vi "Load IV Data.vi"(7 "Other channels":string[](array[string]), 8 "error in":errorcluster, 9 "All scans":refnum<vi>, 10 "Scan numbers":i32[](array[numeric])=[0], 11 "File Path":path=path "U:/My Documents/Projects/Eremets/NV/IV/Data/August_2022/080922/m009_080922.tdms") -> (0 "error out":errorcluster, 1 "dIdV":dbl[](array[numeric]) format="%#_6p", 2 "V":dbl[](array[numeric]), 3 "I":dbl[](array[numeric]), 4 "Other values":string[](array[string]), 5 "Number of scans":i32)   [LabVIEW 2021]
panel:
  out "Numeric 2":i32
  out "Numeric":i32
  out "group names":string[](array[string])
  out "f 2":cluster{dbl[], dbl[]}(graph)
  out "All scans":cluster{dbl[], dbl[]}[](graph)
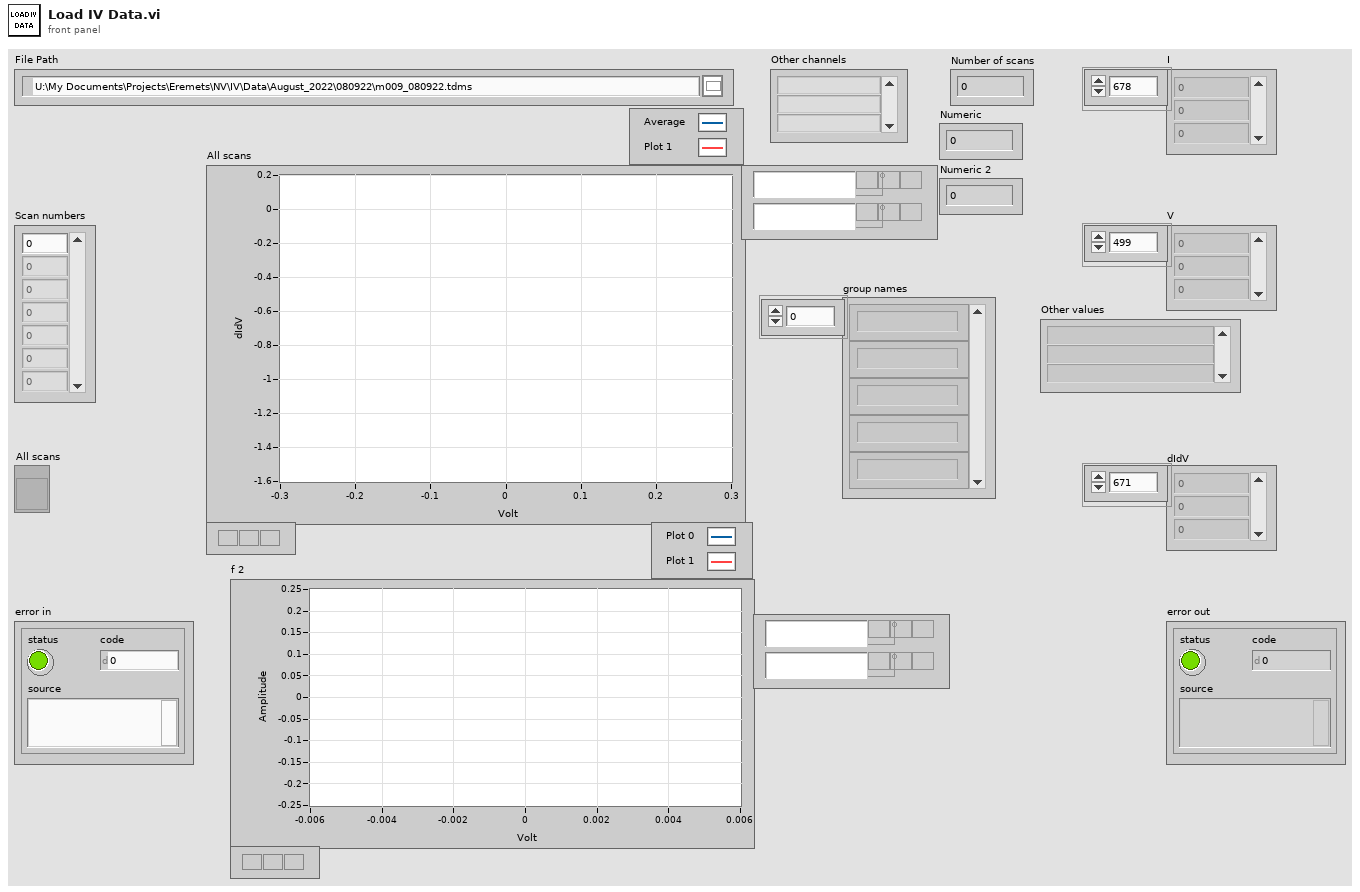
[diagram p1: front panel]
types:
  T1 = enum16{"open", "open or create", "create or replace", "create", "open (read-only)"}
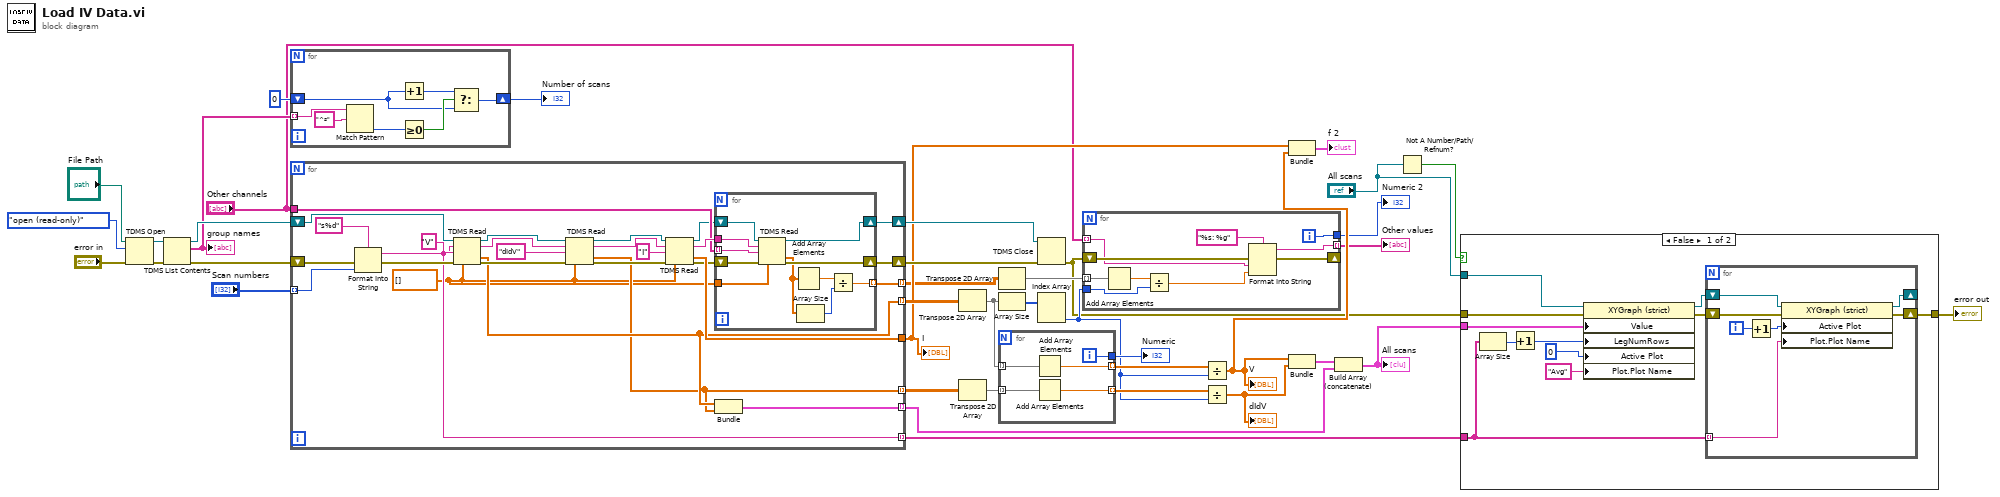
[diagram p0: block diagram]
diagram:
  n1 = TDMS Open(8:"error in", 10:T1."open (read-only)" ("operation (0:open)"), 11:"File Path") -> (0:w18:errorcluster, 3:w20:refnum<k34>)  [unwired: 4 in]
  n2 = TDMS List Contents(4:w18, 7:w20) -> (0:w17:errorcluster, 2:w16:string[], 3:w19:refnum<k34>)  [unwired: 1 in, 1 out]
  "group names" <- w16
  n3 = for {
    tunnel: w16 -> [w46] mode=indexing
    shift-right: [w40] -> w14
    shift-left: 0 -> [w41]
    n4 = Match Pattern(string=w46, regular expression="^s") -> (offset past match=w44:i32)  [unwired: 1 in, 3 out]
    n5 = Increment(x=w41) -> (x+1=w42:i32)
    n6 = Greater Or Equal To 0?(x=w44) -> (x >= 0?=w43:bool)
    n7 = Select(t=w42, s=w43, f=w41) -> (s? t:f=w40:i32)
  }
  "Number of scans" <- w14
  n8 = for {
    shift-right: [w51] -> w35
    shift-left: w17 -> [w64]
    tunnel: [w57] -> w33 mode=indexing
    tunnel: [w67] -> w23
    shift-right: [w49] -> w39
    shift-left: w19 -> [w66]
    tunnel: "Scan numbers" -> [w65] mode=indexing
    tunnel: [w58] -> w31 mode=indexing
    tunnel: [w56] -> w30 mode=indexing
    tunnel: [w55] -> w10 mode=indexing
    tunnel: "Other channels" -> [w53]
    tunnel: [w47] -> w8 mode=indexing
    w48 = dbl[] []
    n9 = Format Into String(format string="s%d", error in=w64, w65) -> (resulting string=w55:string, error out=w63:errorcluster)  [unwired: 1 in]
    n10 = TDMS Read(0:w66, 5:w55, 7:"V", 11:w63, 12:w48) -> (4:w73:refnum<k34>, 6:w72:string, 10:w58:dbl[], 15:w71:errorcluster)  [unwired: 3 in, 2 out]
    n11 = TDMS Read(0:w73, 5:w72, 7:"dIdV", 11:w71, 12:w48) -> (4:w69:refnum<k34>, 6:w68:string, 10:w57:dbl[], 15:w70:errorcluster)  [unwired: 3 in, 2 out]
    n12 = TDMS Read(0:w69, 5:w68, 7:"I", 11:w70, 12:w48) -> (4:w50:refnum<k34>, 6:w54:string, 10:w67:dbl[], 15:w52:errorcluster)  [unwired: 3 in, 2 out]
    n13 = for {
      tunnel: w54 -> [w84]
      tunnel: w53 -> [w83] mode=indexing
      shift-right: [w81] -> w51
      shift-left: w52 -> [w82]
      shift-right: [w79] -> w49
      shift-left: w50 -> [w80]
      tunnel: w48 -> [w78]
      tunnel: [w74] -> w47 mode=indexing
      n14 = TDMS Read(0:w80, 5:w84, 7:w83, 11:w82, 12:w78) -> (4:w79:refnum<k34>, 10:w77:dbl[], 15:w81:errorcluster)  [unwired: 3 in, 3 out]
      n15 = Add Array Elements(numeric array=w77) -> (sum=w76:dbl)
      n16 = Array Size(array=w77) -> (size(s)=w75:i32)
      n17 = Divide(x=w76, y=w75) -> (x/y=w74:dbl)
    }
    n18 = Bundle(w58, w57) -> (w56:cluster{dbl[], dbl[]})  [unwired: 1 in]
  }
  "I" <- w23
  n19 = Transpose 2D Array(2D array=w31) -> (transposed array=w25:dbl[][])
  n20 = Transpose 2D Array(2D array=w33) -> (transposed array=w32:dbl[][])
  n21 = Transpose 2D Array(2D array=w8) -> (transposed array=w6:dbl[][])
  n22 = Array Size(array=w25) -> (size(s)=w24:i32[])
  n23 = for {
    tunnel: w32 -> [w89] mode=indexing
    tunnel: [w88] -> w26 mode=indexing
    tunnel: w25 -> [w87] mode=indexing
    tunnel: [w86] -> w28 mode=indexing
    tunnel: [w85] -> w7
    i -> [w85]
    n24 = Add Array Elements(numeric array=w87) -> (sum=w86:dbl)
    n25 = Add Array Elements(numeric array=w89) -> (sum=w88:dbl)
  }
  "Numeric" <- w7
  n26 = TDMS Close(8:w35, 11:w39) -> (0:w3:errorcluster)  [unwired: 1 out]
  n27 = Index Array(array=w24) -> (element #2=w4:i32)  [unwired: 2 in, 1 out]
  n28 = for {
    tunnel: w6 -> [w99] mode=indexing
    tunnel: [w98] -> w5
    tunnel: w4 -> [w97]
    shift-right: [w94] -> _
    shift-left: w3 -> [w95]
    tunnel: "Other channels" -> [w91] mode=indexing
    tunnel: [w90] -> w1 mode=indexing
    i -> [w98]
    n29 = Add Array Elements(numeric array=w99) -> (sum=w96:dbl)
    n30 = Divide(x=w96, y=w97) -> (x/y=w92:dbl)
    n31 = Format Into String(format string="%s: %g", error in=w95, w91, w92) -> (resulting string=w90:string, error out=w94:errorcluster)  [unwired: 1 in]
  }
  "Numeric 2" <- w5
  "Other values" <- w1
  n32 = Divide(x=w28, y=w4) -> (x/y=w22:dbl[])
  "V" <- w22
  n33 = Divide(x=w26, y=w4) -> (x/y=w27:dbl[])
  "dIdV" <- w27
  n34 = Bundle(w23, w22) -> (→"f 2":cluster{dbl[], dbl[]})  [unwired: 1 in]
  n35 = Bundle(w22, w27) -> (w29:cluster{dbl[], dbl[]})  [unwired: 1 in]
  n36 = Build Array (concatenate)(w29, w30) -> (w11:cluster{dbl[], dbl[]}[])
  "All scans" <- w11
  n37 = Not A Number/Path/Refnum?(number/path/refnum="All scans") -> (NaN/Path/Refnum?=w13:bool)
  n38 = case shown="False" w13 {
    tunnel: "All scans" -> [w110 _]
    tunnel: w11 -> [w109 _]
    tunnel: w3 -> [w108 w118]
    tunnel: w10 -> [w102 _]
    tunnel: [w103 w118] -> w9
    frame False {
      n39 = Array Size(array=w102) -> (size(s)=w101:i32)
      n40 = Increment(x=w101) -> (x+1=w100:i32)
      n41 = property class="XYGraph (strict)"(reference=w110, error in=w108, "Value"=w109, "LegNumRows"=w100, "Active Plot"=u32 0, "Plot.Plot Name"="Avg") -> (reference out=w107:refnum<vi>, error out=w104:errorcluster)
      n42 = for {
        tunnel: w102 -> [w116] mode=indexing
        shift-right: [w113] -> _
        shift-left: w107 -> [w114]
        shift-right: [w111] -> w103
        shift-left: w104 -> [w112]
        i -> [w117]
        n43 = Increment(x=w117) -> (x+1=w115:i32)
        n44 = property class="XYGraph (strict)"(reference=w114, error in=w112, "Active Plot"=w115, "Plot.Plot Name"=w116) -> (reference out=w113:refnum<vi>, error out=w111:errorcluster)
      }
    }
    frame True {
    }
  }
  "error out" <- w9
